vi "Str.vi"(4 "String":string) -> (1 "Abs_String.lvclass":refnum<class "Abs_String.lvclass">)   [LabVIEW 2021, in "Const_Str.lvclass"]
uses:
  Const_Str.lvclass
  Abs_Types/String/Abs_String.lvclass
  C:/Program Files (x86)/National Instruments/LabVIEW 2021/vi.lib/TSA/Abstract Data Classes/Abs_Types/String/Abs_String.lvclass
  Const_Str.lvclass/Const_Str.ctl
  Properties/Write Value.vi
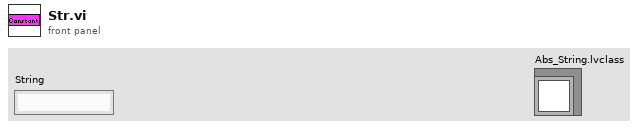
[diagram p1: front panel]
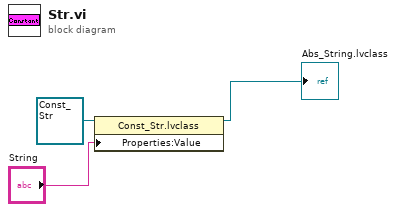
[diagram p0: block diagram]
diagram:
  n1 = property class="Const_Str.lvclass"(reference=refnum<class "Const_Str.lvclass"> refnum ("Const_Str.lvclass"), "Properties:Value"="String") -> (reference out=→"Abs_String.lvclass":refnum<class "Const_Str.lvclass">)  [unwired: 1 in, 1 out]
